vi "ths_browser_comparator_mpix.vi"() -> ()   [LabVIEW 2021]
panel:
  in  "file B":path=path "C:/scan/thscan.bin"
  in  "file A":path=path "C:/scan/thscan.bin"
  out "MainImg":u16[][](graph)
  out "Th Scan":u16[][](graph)
  in  "ThScan_Load":bool
  out "ThScan":i32[][][](array[numeric])
  in  "Exit":bool
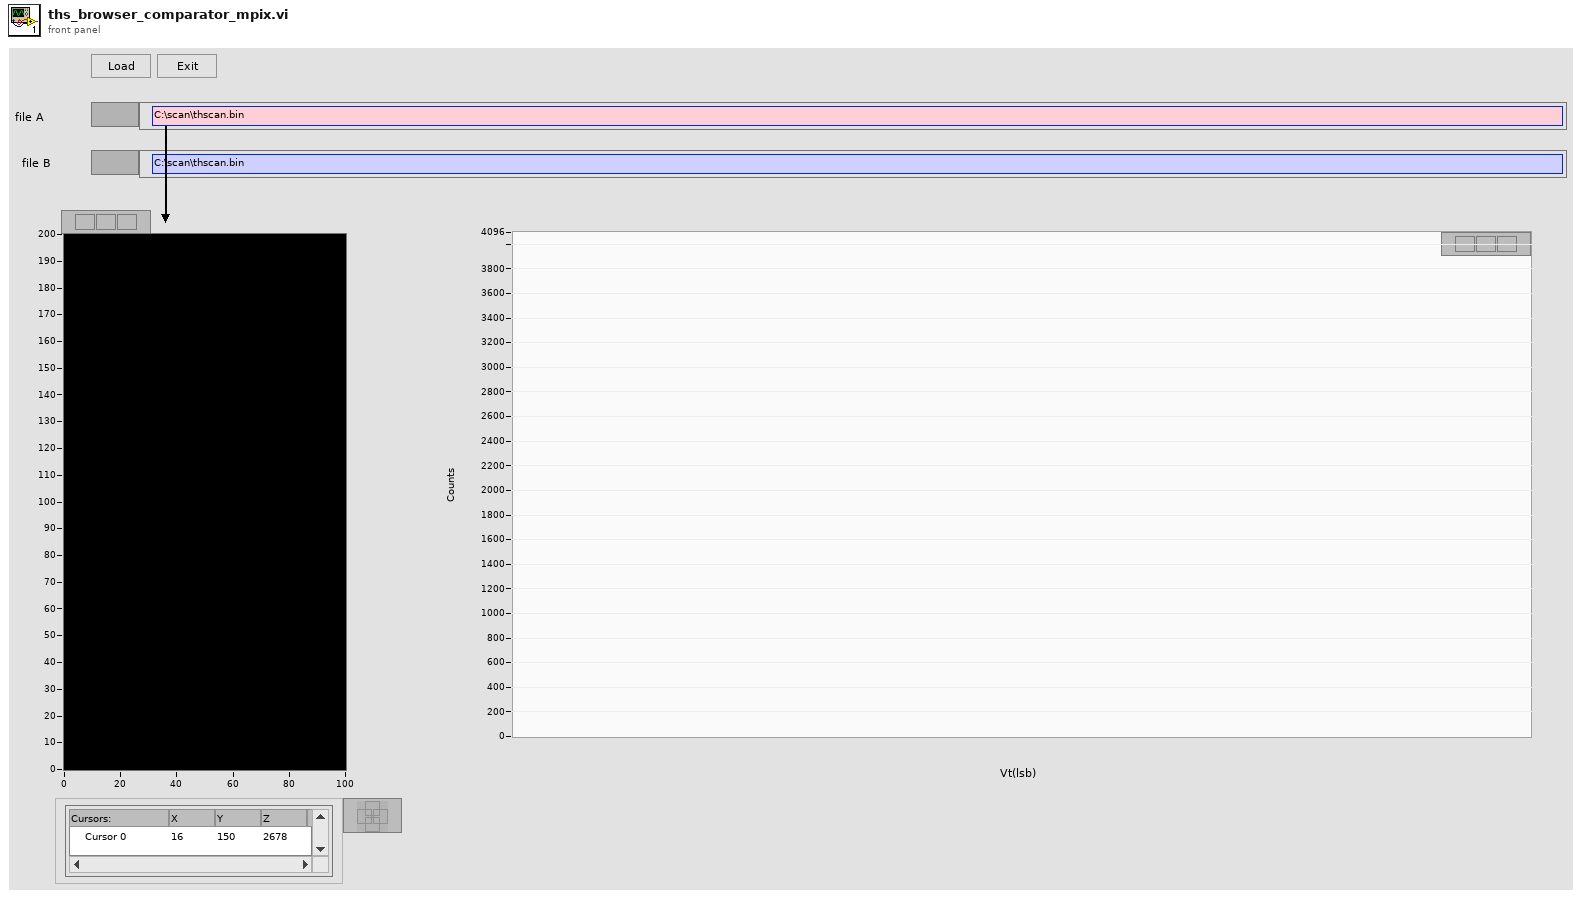
[diagram p1: front panel]
types:
  T1 = enum16{"big-endian, network order", "native, host order", "little-endian"}
  T2 = typedef "LVPointDoubleTypeDef.ctl" = cluster{"Cursor X":dbl, "Cursor Y":dbl}
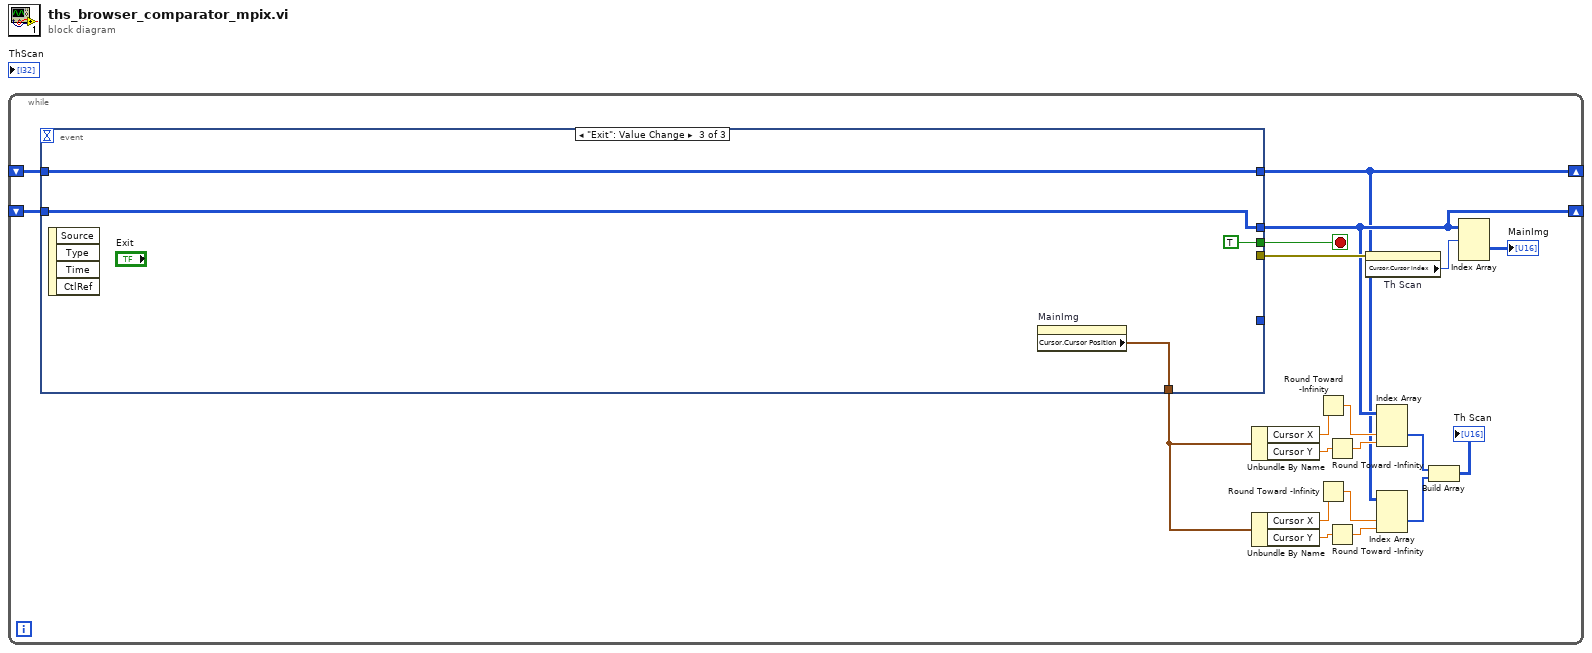
[diagram p0: block diagram]
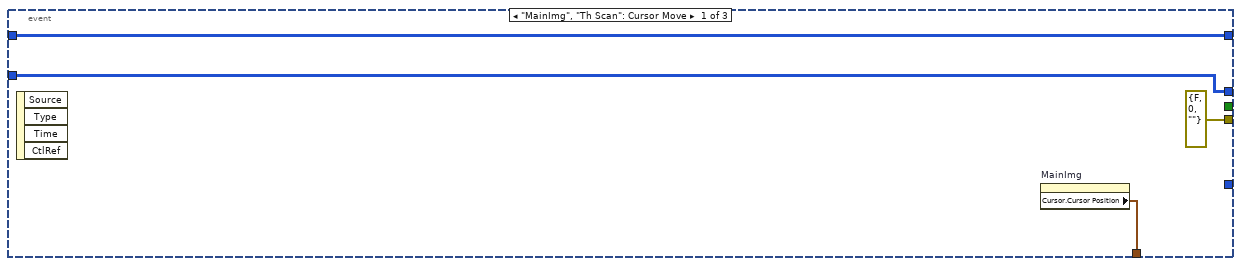
[diagram p2: hidden frame]
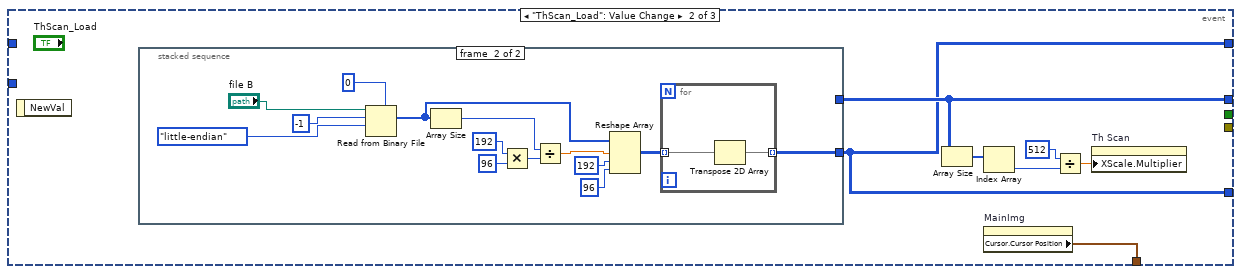
[diagram p3: hidden frame]
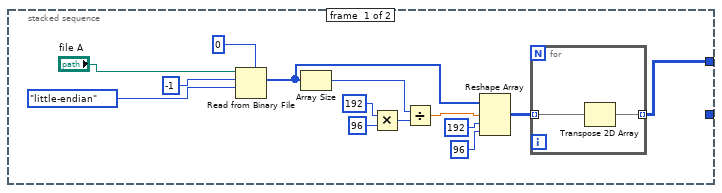
[diagram p4: hidden frame]
diagram:
  n1 = while {
    shift-right: [w16] -> _
    shift-left: _ -> [w15]
    shift-right: [w1] -> _
    shift-left: _ -> [w2]
    stop <- w20 stop-if-true
    n2 = event shown="[2] \"Exit\": Value Change" {
      selector: _ -> [_ _ _]
      dyn-events: _ -> [_ _ _]
      timeout: _ -> [_ _ _]
      tunnel: [_ _ TRUE] -> w20
      tunnel: [errorcluster {"status"=FALSE, "code"=0, "source"=""} ("error in (no error)") _ _] -> w17
      tunnel: w15 -> [w23 _ w66]
      tunnel: [w23 w31 w66] -> w16
      tunnel: [w22 w30 w65] -> w6
      tunnel: [_ w25 _] -> _
      tunnel: [w21 w25 w64] -> w1
      tunnel: w2 -> [w21 _ w64]
      event "MainImg", "Th Scan": Cursor Move {
        n3 = event-data() -> ()  [unwired: 1 in, 4 out]
        n4 = property on="MainImg" class="IntGraph (strict)"() -> ("Cursor.Cursor Position"=w22:T2)  [unwired: 2 in, 2 out]
      }
      event "ThScan_Load": Value Change {
        n5 = event-data() -> ()  [unwired: 1 in, 1 out]
        n6 = stacked-sequence {
          tunnel: [w45 _] -> w31
          tunnel: [_ w49] -> w25
          frame #0 {
            n7 = Read from Binary File(5:u16 0, 9:T1."little-endian" ("byte order (0:big-endian, network order)"), 10:-1 ("count (1)"), 11:"file A") -> (2:w34:u16[])  [unwired: 2 in, 3 out]
            n8 = Array Size(array=w34) -> (size(s)=w39:i32)
            n9 = Multiply(x=192 ("dimension size"), y=96 ("dimension size")) -> (x*y=w36:i32)
            n10 = Divide(x=w39, y=w36) -> (x/y=w35:dbl)
            n11 = Reshape Array(w34, w35, 192 ("dimension size"), 96 ("dimension size")) -> (w33:u16[][][])
            n12 = for {
              tunnel: w33 -> [w47] mode=indexing
              tunnel: [w46] -> w45 mode=indexing
              n13 = Transpose 2D Array(2D array=w47) -> (transposed array=w46:u16[][])
            }
          }
          frame #1 {
            n14 = Read from Binary File(5:u16 0, 9:T1."little-endian" ("byte order (0:big-endian, network order)"), 10:-1 ("count (1)"), 11:"file B") -> (2:w51:u16[])  [unwired: 2 in, 3 out]
            n15 = Array Size(array=w51) -> (size(s)=w56:i32)
            n16 = Multiply(x=192 ("dimension size"), y=96 ("dimension size")) -> (x*y=w53:i32)
            n17 = Divide(x=w56, y=w53) -> (x/y=w52:dbl)
            n18 = Reshape Array(w51, w52, 192 ("dimension size"), 96 ("dimension size")) -> (w50:u16[][][])
            n19 = for {
              tunnel: w50 -> [w63] mode=indexing
              tunnel: [w62] -> w49 mode=indexing
              n20 = Transpose 2D Array(2D array=w63) -> (transposed array=w62:u16[][])
            }
          }
        }
        n21 = Array Size(array=w31) -> (size(s)=w29:i32[])
        n22 = Index Array(array=w29) -> (element=w28:i32)  [unwired: 1 in]
        n23 = property on="MainImg" class="IntGraph (strict)"() -> ("Cursor.Cursor Position"=w30:T2)  [unwired: 2 in, 2 out]
        n24 = Divide(x=512, y=w28) -> (x/y=w26:dbl)
        n25 = property on="Th Scan" class="WFGraph (strict)"("XScale.Multiplier"=w26) -> ()  [unwired: 2 in, 2 out]
      }
      event "Exit": Value Change {
        n26 = event-data() -> ()  [unwired: 1 in, 4 out]
        n27 = property on="MainImg" class="IntGraph (strict)"() -> ("Cursor.Cursor Position"=w65:T2)  [unwired: 2 in, 2 out]
      }
    }
    n28 = Unbundle By Name(w6) -> ("Cursor X"=w12:dbl, "Cursor Y"=w13:dbl)
    n29 = Unbundle By Name(w6) -> ("Cursor X"=w8:dbl, "Cursor Y"=w9:dbl)
    n30 = Round Toward -Infinity(1:w12) -> (0:w11:dbl)
    n31 = Round Toward -Infinity(1:w8) -> (0:w7:dbl)
    n32 = Round Toward -Infinity(1:w13) -> (0:w14:dbl)
    n33 = Round Toward -Infinity(1:w9) -> (0:w10:dbl)
    n34 = property on="Th Scan" class="WFGraph (strict)"(error in=w17) -> ("Cursor.Cursor Index"=w18:i32)  [unwired: 1 in, 2 out]
    n35 = Index Array(array=w16, index (dim 1)=w11, index (dim 2)=w14) -> (element=w5:u16[])  [unwired: 1 in]
    n36 = Index Array(array=w1, index (dim 1)=w7, index (dim 2)=w10) -> (element=w4:u16[])  [unwired: 1 in]
    n37 = Build Array(w5, w4) -> (→"Th Scan":u16[][])
    n38 = Index Array(array=w16, index (dim 0)=w18) -> (element=→"MainImg":u16[][])  [unwired: 2 in]
  }
